vi "getCameraSettingsPath.vi"(8 "error in (no error)":errorcluster, 10 "Camera":enum16{"Pixis", "ProEM", "PixelFly"}(ring), 11 "FileSystem.lvclass in":refnum<class "FileSystem.lvclass">) -> (0 "error out":errorcluster, 2 "CameraSettingsPath":path, 3 "FileSystem.lvclass out":refnum<class "FileSystem.lvclass">)   [LabVIEW 2011, in "Tools.lvlib" / "Filing.lvlib" / "FileSystem.lvclass"]
uses:
  FileSystem.lvclass
  FileSystem.lvclass/FileSystem.ctl
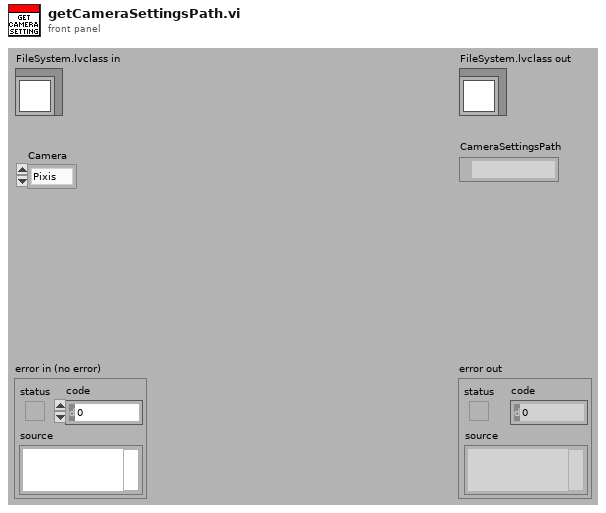
[diagram p1: front panel]
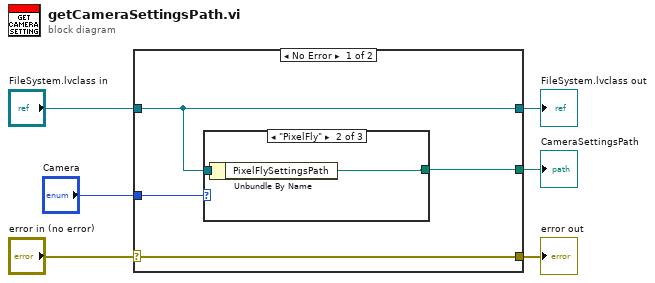
[diagram p0: block diagram]
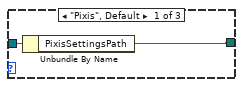
[diagram p2: hidden frame]
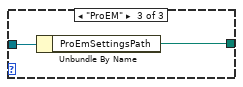
[diagram p3: hidden frame]
diagram:
  n1 = case shown="No Error" "error in (no error)" {
    selector: "error in (no error)" -> [w10 w17]
    tunnel: [w10 w17] -> w5
    tunnel: [w9 w18] -> w3
    tunnel: "FileSystem.lvclass in" -> [w9 w18]
    tunnel: [w8 _] -> w2
    tunnel: "Camera" -> [w7 _]
    frame No Error {
      n2 = case shown="\"PixelFly\"" w7 {
        tunnel: w9 -> [w12 w14 w16]
        tunnel: [w11 w13 w15] -> w8
        frame "Pixis", Default {
          n3 = Unbundle By Name(w12) -> ("PixisSettingsPath"=w11:path)
        }
        frame "PixelFly" {
          n4 = Unbundle By Name(w14) -> ("PixelFlySettingsPath"=w13:path)
        }
        frame "ProEM" {
          n5 = Unbundle By Name(w16) -> ("ProEmSettingsPath"=w15:path)
        }
      }
    }
    frame Error {
    }
  }
  "error out" <- w5
  "FileSystem.lvclass out" <- w3
  "CameraSettingsPath" <- w2
